vi "Get Goal.vi"() -> (2 "Left Goal?":bool, 6 "Robot Relative X (Target)":dbl, 8 "Robot Relative Y (Target)":dbl, 10 "Camera Relative X (Target)":dbl, 12 "Field-Rel VisTarget X":dbl, 13 "Target Distance":dbl, 14 "Goal Found?":bool, 15 "Camera Relative Y (Target)":dbl)   [LabVIEW 2013]
uses:
  Robot Global Data.vi
panel:
  # "Angle to the tracking tape\n(not the center of the goal)"
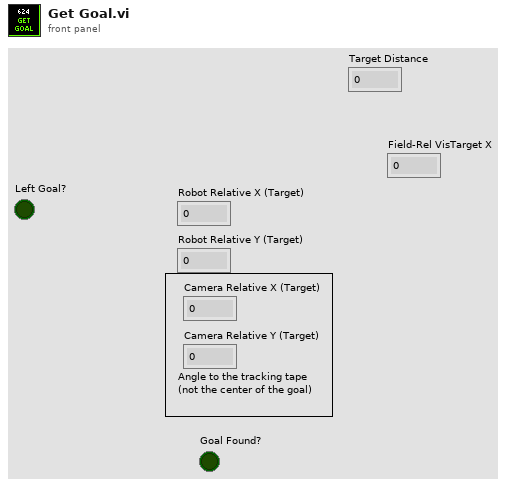
[diagram p1: front panel]
types:
  T1 = typedef "Vision Packet.ctl" = cluster{"Gyro":dbl, "Vision Target":T2, "Timestamp":u32, "Left Goal":T2, "Right Goal":T2}
  T2 = typedef "Goal Info.ctl" = cluster{"Found?":bool, "Target Center":cluster{"X":dbl, "Y":dbl}, "Distance (ft)":dbl, "Hot?":bool, "Left?":bool, "Camera":i16}
  T3 = typedef "Dashboard UDP Packet.ctl" = cluster{"Camera":T4, "Gyro":T5, "Encoder":T6, "Auto Shift":T7, "Auton":T8, "Drive/Ramp X":dbl, "Drive/Ramp Y":dbl, "Drive/Battery Cutoff":dbl, "Pressure/Compressor Min Voltage":dbl, "Pressure/Compressor Delay":dbl, "Controller/Strafe Correction":bool, "Shooter":T9, "Rollers":T10, "Abort":bool, "Finish":bool}
  T4 = typedef "Camera Controls.ctl" = cluster{"Camera/View Angle X":dbl, "Camera/Goal Track Timeout":dbl, "Camera/View Angle Y":dbl, "Camera/Goal Exposure":dbl, "Camera/Vision Receive Timeout":dbl, "Camera/Offset 1":dbl, "Camera/Offset 2":dbl}
  T5 = typedef "Gyro Controls.ctl" = cluster{"Gyro/Steer Close PID P":dbl, "Gyro/Steer Close PID I":dbl, "Gyro/Steer Close PID D":dbl, "Gyro/Steer Close PID min":dbl, "Gyro/Steer Close PID max":dbl, "Gyro/Steer PID P":dbl, "Gyro/Steer PID I":dbl, "Gyro/Steer PID D":dbl, "Gyro/Steer PID min":dbl, "Gyro/Angle Tolerance":dbl, "Gyro/Steer PID max":dbl, "Gyro/Steer Closeness Threshold":dbl}
  T6 = typedef "Encoder Controls.ctl" = cluster{"Encoders/Reset":bool, "Encoders/Omni Constant":dbl, "Encoders/Omni Tick Constant":dbl, "Encoders/Left Constant":dbl, "Encoders/Right Constant":dbl, "Encoders/Right Tick Constant":dbl}
  T7 = typedef "Auto Shift Controls.ctl" = cluster{"AutoShift/Upshift Throttle Accel":dbl, "AutoShift/Speed Threshold":dbl, "AutoShift/Upshift Throttle":dbl, "AutoShift/Upshift Accel":dbl, "AutoShift/Downshift Accel":dbl, "AutoShift/Downshift Throttle":dbl, "AutoShift/Delay":dbl, "AutoShift/Enabled":bool}
  T8 = typedef "Auton Controls.ctl" = cluster{"Auton/Left Shoot X-Coord":dbl, "Auton/Right Shoot X-Coord":dbl, "DistDrive/Distance Stop Threshold":dbl, "DistDrive/Max Stop Speed":dbl, "Auton/Back Piston Time":dbl, "Auton/Manual Hot":bool, "Auton/Manual Hot Right":bool, "Auton/X Distance PID max":dbl, "Auton/X Distance PID min":dbl, "Auton/X Distance PID P":dbl, "Auton/X Distance PID I":dbl, "Auton/X Distance PID D":dbl, "Auton/Y Distance PID max":dbl, "Auton/Y Distance PID min":dbl, "Auton/Y Distance PID P":dbl, "Auton/Y Distance PID I":dbl, "Auton/Y Distance PID D":dbl}
  T9 = typedef "Shooter Controls.ctl" = cluster{"Shooter/Reset Time":dbl, "Shooter/Release Delay":dbl, "Shooter/Pressure Steady Time":dbl, "Shooter/Misfire Delay":dbl, "Shooter/Ball Settle Time":dbl, "Shooter/Line IR Delay":dbl, "Pressure/Upper PSI Time":dbl, "Pressure/Lower PSI Time":dbl, "Shooter/Punch Delay":dbl, "Shooter/Target Pressure":dbl, "Pressure/Line B":dbl, "Pressure/Line M":dbl, "Pressure/Shooter M":dbl, "Pressure/Shooter B":dbl}
  T10 = typedef "Roller Controls.ctl" = cluster{"Roller/Load IRs Verify Time":dbl, "Roller/Center IR Latch Time":dbl, "Roller/Speed Front":dbl, "Roller/Speed Back":dbl, "Roller/Entry Timeout":dbl, "Roller/To Center Timeout":dbl, "Roller/Sustain Time":dbl, "Roller/Verify Center Time":dbl}
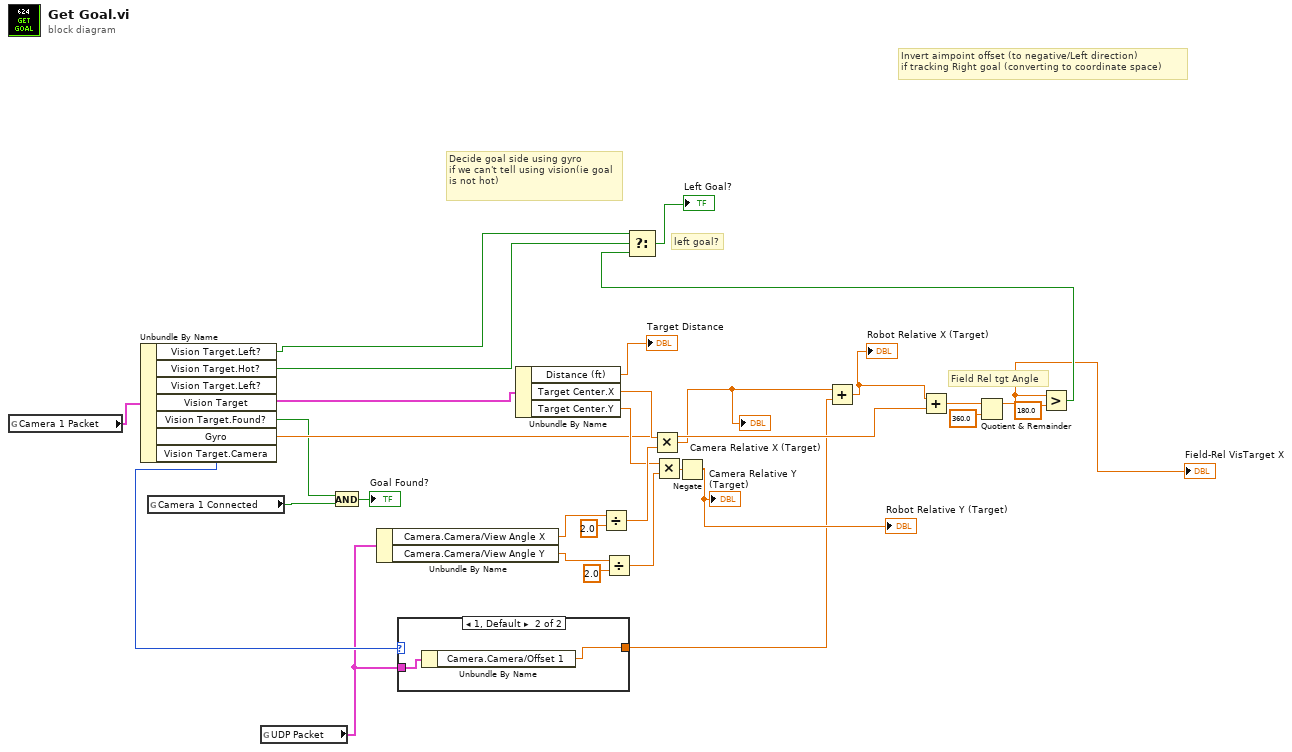
[diagram p0: block diagram]
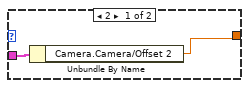
[diagram p2: hidden frame]
diagram:
  # "Decide goal side using gyro\nif we can't tell using vision(ie goal is not hot)"
  # "left goal?"
  # "Field Rel tgt Angle"
  # "Invert aimpoint offset (to negative/Left direction)\nif tracking Right goal (converting to coordinate space)"
  n1 = global read "Robot Global Data.vi" "Camera 1 Packet"() -> (w22:T1)
  n2 = Unbundle By Name(w22) -> ("Vision Target.Left?"=w12:bool, "Vision Target.Hot?"=w10:bool, "Vision Target"=w15:T2, "Vision Target.Found?"=w16:bool, "Gyro"=w17:dbl, "Vision Target.Camera"=w7:i16)  [unwired: 1 out]
  n3 = global read "Robot Global Data.vi" "Camera 1 Connected"() -> (w25:bool)
  n4 = global read "Robot Global Data.vi" "UDP Packet"() -> (w1:T3)
  n5 = And(x=w16, y=w25) -> (x .and. y?=→"Goal Found?":bool)
  n6 = Unbundle By Name(w1) -> ("Camera.Camera/View Angle X"=w3:dbl, "Camera.Camera/View Angle Y"=w2:dbl)
  n7 = case shown="1, Default" w7 {
    tunnel: [w31 w33] -> w5
    tunnel: w1 -> [w32 w34]
    frame 2 {
      n8 = Unbundle By Name(w32) -> ("Camera.Camera/Offset 2"=w31:dbl)
    }
    frame 1, Default {
      n9 = Unbundle By Name(w34) -> ("Camera.Camera/Offset 1"=w33:dbl)
    }
  }
  n10 = Unbundle By Name(w15) -> ("Distance (ft)"=→"Target Distance":dbl, "Target Center.X"=w20:dbl, "Target Center.Y"=w19:dbl)
  n11 = Divide(x=w3, y=2.0) -> (x/y=w28:dbl)
  n12 = Divide(x=w2, y=2.0) -> (x/y=w27:dbl)
  n13 = Multiply(x=w20, y=w28) -> (x*y=w6:dbl)
  "Camera Relative X (Target)" <- w6
  n14 = Multiply(x=w19, y=w27) -> (x*y=w26:dbl)
  n15 = Negate(x=w26) -> (-x=→"Robot Relative Y (Target)" →"Camera Relative Y (Target)":dbl)
  n16 = Add(x=w6, y=w5) -> (x+y=w4:dbl)
  "Robot Relative X (Target)" <- w4
  n17 = Add(x=w4, y=w17) -> (x+y=w24:dbl)
  n18 = Quotient & Remainder(x=w24, y=360.0) -> (x-y*floor(x/y)=w9:dbl)  [unwired: 1 out]
  "Field-Rel VisTarget X" <- w9
  n19 = Greater?(x=w9, y=180.0) -> (0:w13:bool)
  n20 = Select(t=w12, s=w10, f=w13) -> (s? t:f=→"Left Goal?":bool)
